vi "PatientProgress.vi"() -> ()   [LabVIEW 2013, in "main.lvlib"]
uses:
  main.lvlib
panel:
  out "Array":i32[][](array[numeric])
  in  "PatientID":path
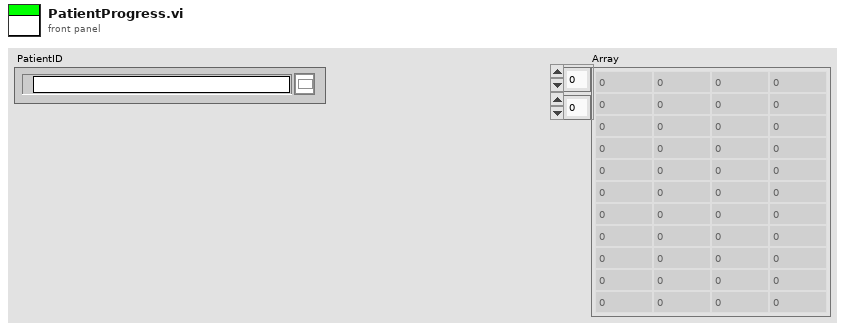
[diagram p1: front panel]
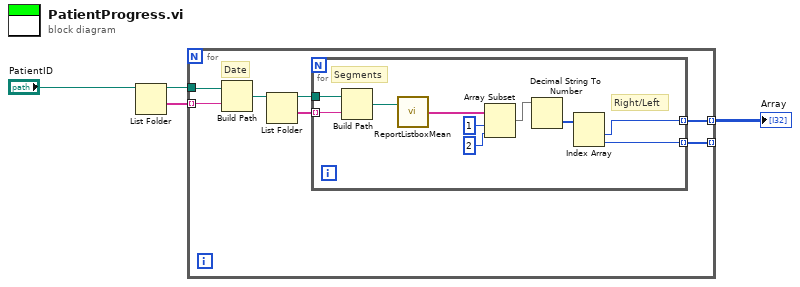
[diagram p0: block diagram]
diagram:
  n1 = List Folder(path="PatientID") -> (path out=w2:path, folder names=w3:string[])  [unwired: 3 in, 2 out]
  n2 = for {
    tunnel: w3 -> [w10] mode=indexing
    tunnel: w2 -> [w11]
    tunnel: [w6] -> w1 mode=indexing
    tunnel: [w5] -> _ mode=indexing
    # "Date"
    n3 = Build Path(base path=w11, name or relative path=w10) -> (appended path=w9:path)
    n4 = List Folder(path=w9) -> (path out=w8:path, folder names=w7:string[])  [unwired: 3 in, 2 out]
    n5 = for {
      tunnel: w8 -> [w20]
      tunnel: w7 -> [w21] mode=indexing
      tunnel: [w13] -> w6 mode=indexing
      tunnel: [w12] -> w5 mode=indexing
      # "Right/Left"
      # "Segments"
      n6 = Build Path(base path=w20, name or relative path=w21) -> (appended path=w19:path)
      n7 = call "ReportListboxMean.vi"("path"=w19) -> ("Means"=w18:string[])  [unwired: 1 in, 2 out]
      n8 = Array Subset(array=w18, index=1, length=2) -> (w15:string[])
      n9 = Decimal String To Number(string=w15) -> (number=w14:i32[])  [unwired: 2 in, 1 out]
      n10 = Index Array(array=w14) -> (element #1=w13:i32, element #2=w12:i32)  [unwired: 2 in]
    }
  }
  "Array" <- w1
